vi "Calc.vi"(11 "Commands":T3) -> (3 "Outputs":T1)   [LabVIEW 2012]
uses:
  util/Commands.ctl
  climber/climber_cmds.ctl
  util/Outputs.ctl
  climber/climber_outputs.ctl
panel:
  in  "Outputs 2":T1
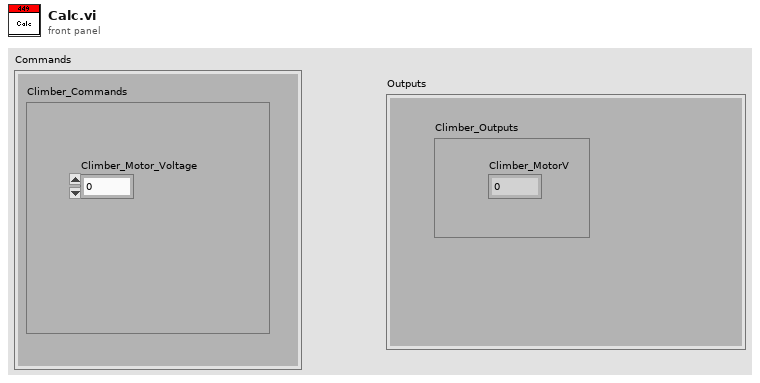
[diagram p1: front panel]
types:
  T1 = typedef "Outputs.ctl" = cluster{"Climber_Outputs":T2}
  T2 = typedef "climber_outputs.ctl" = cluster{"Climber_MotorV":dbl}
  T3 = typedef "Commands.ctl" = cluster{"Climber_Commands":T4}
  T4 = typedef "climber_cmds.ctl" = cluster{"Climber_Motor_Voltage":dbl}
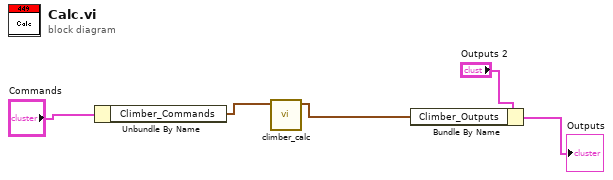
[diagram p0: block diagram]
diagram:
  n1 = Unbundle By Name("Commands") -> ("Climber_Commands"=w4:T4)
  n2 = call "climber_calc.vi"("Climber_Commands"=w4) -> ("Climber_Outputs"=w1:T2)  [unwired: 10 in]
  n3 = Bundle By Name(cluster="Outputs 2", "Climber_Outputs"=w1) -> (→"Outputs":T1)
